vi "17_ВПОсциллограф.vi"() -> ()   [LabVIEW 2016]
panel:
  in  "Boolean":bool
  out "Waveform Chart":dbl(graph)
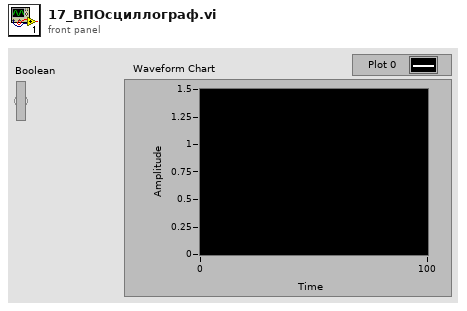
[diagram p1: front panel]
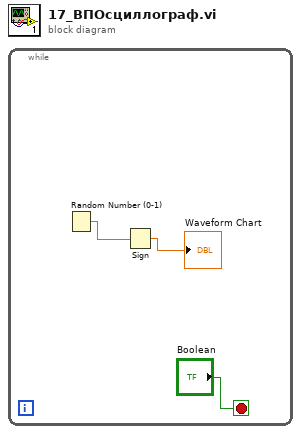
[diagram p0: block diagram]
diagram:
  n1 = while {
    stop <- "Boolean" stop-if-true
    n2 = Random Number (0-1)() -> (number: 0 to 1=w1:dbl)
    n3 = Sign(1:w1) -> (0:→"Waveform Chart":dbl)
  }
